vi "SnapToScore.vi"(7 "PigeonIMUDevRef":T1={"DeviceStatus"={"status"=FALSE, "code"=0, "source"=""}, "Device Number"=0, "Type"=352321536, "Device ID"=0, "Handle"=0, "UsageFrame"=0, "Library Path"=path ""} {"Type" items=["CAN"=352321536, "TalonSRX"=33554432]}, 11 "Robot Velocities In":cluster{"x":dbl, "y":dbl, "w":dbl}) -> (3 "Robot Velocities Out":cluster{"x":dbl, "y":dbl, "w":dbl})   [LabVIEW 2020]
uses:
  <vilib>/Rock Robotics/WPI/ThirdParty/Phoenix-LabVIEW/Pigeon IMU/CTRE_PigeonIMU_DeviceRef.ctl
  <vilib>/Rock Robotics/WPI/ThirdParty/Phoenix-LabVIEW/Pigeon IMU/CTRE_PigeonIMU_ConnectionType.ctl
  <vilib>/Analysis/coordinate.llb/Angle Range (Degree).ctl
  <vilib>/Analysis/coordinate.llb/Angle Units.ctl
  <vilib>/Analysis/_algsub.llb/Real Vector Norm.vi
  <vilib>/Analysis/coordinate.llb/Wrap Angle (scalar).vi
  <vilib>/Rock Robotics/WPI/ThirdParty/Phoenix-LabVIEW/Pigeon IMU/CTRE_PigeonIMU_GetYPR.vi
  <vilib>/Analysis/NI_AAL_Angle.lvlib
  <vilib>/Analysis/NI_AALPro.lvlib
panel:
  in  "Precision (deg)":dbl=0.25
  in  "static threshold":dbl=1.55
  in  "FEEEED":dbl=6.6
  out "Err/Out Chart":cluster{dbl, dbl}(graph)
  out "SP/PV Chart":cluster{"setpoint":dbl, "process variable":dbl}(graph)
  out "angle error":dbl
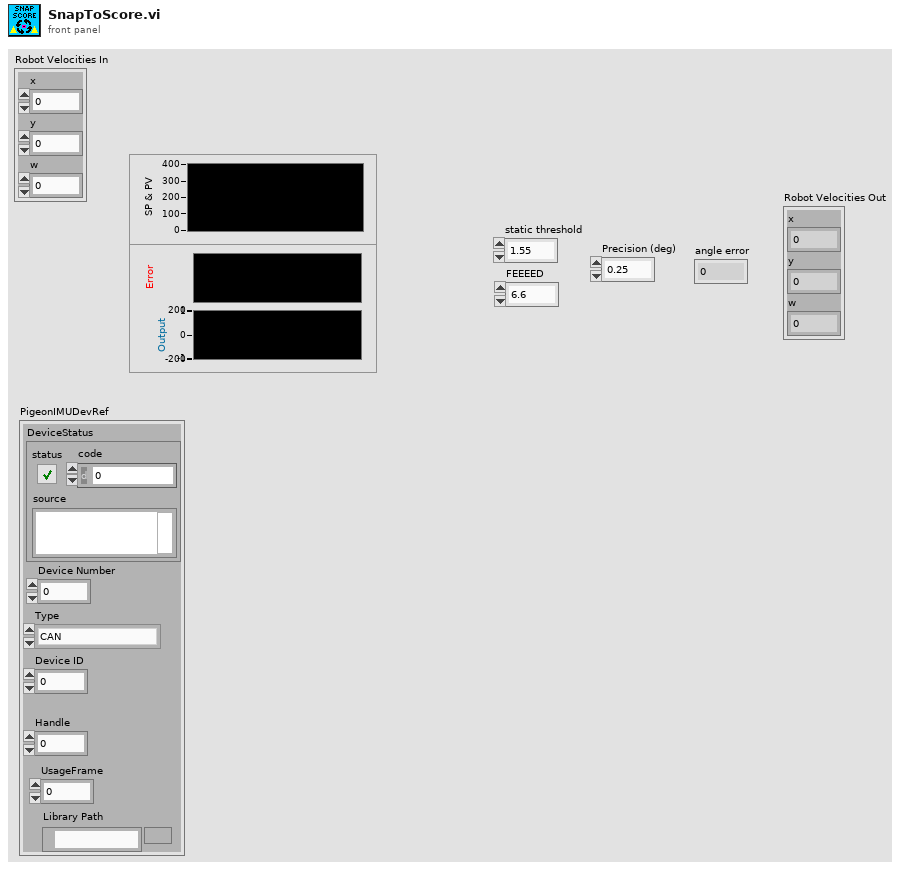
[diagram p1: front panel]
types:
  T1 = typedef "CTRE_PigeonIMU_DeviceRef.ctl" = cluster{"DeviceStatus":errorcluster, "Device Number":u8, "Type":T2, "Device ID":u32, "Handle":u64, "UsageFrame":u32, "Library Path":path}
  T2 = typedef "CTRE_PigeonIMU_ConnectionType.ctl" = u32
  T3 = cluster{"proportional gain (Kp)":dbl, "integral time (Ki)":dbl, "derivative time (Kd)":dbl}
  T4 = typedef "NI_AAL_Angle.lvlib/Angle Units.ctl" = i32
  T5 = typedef "NI_AAL_Angle.lvlib/Angle Range (Degree).ctl" = u16
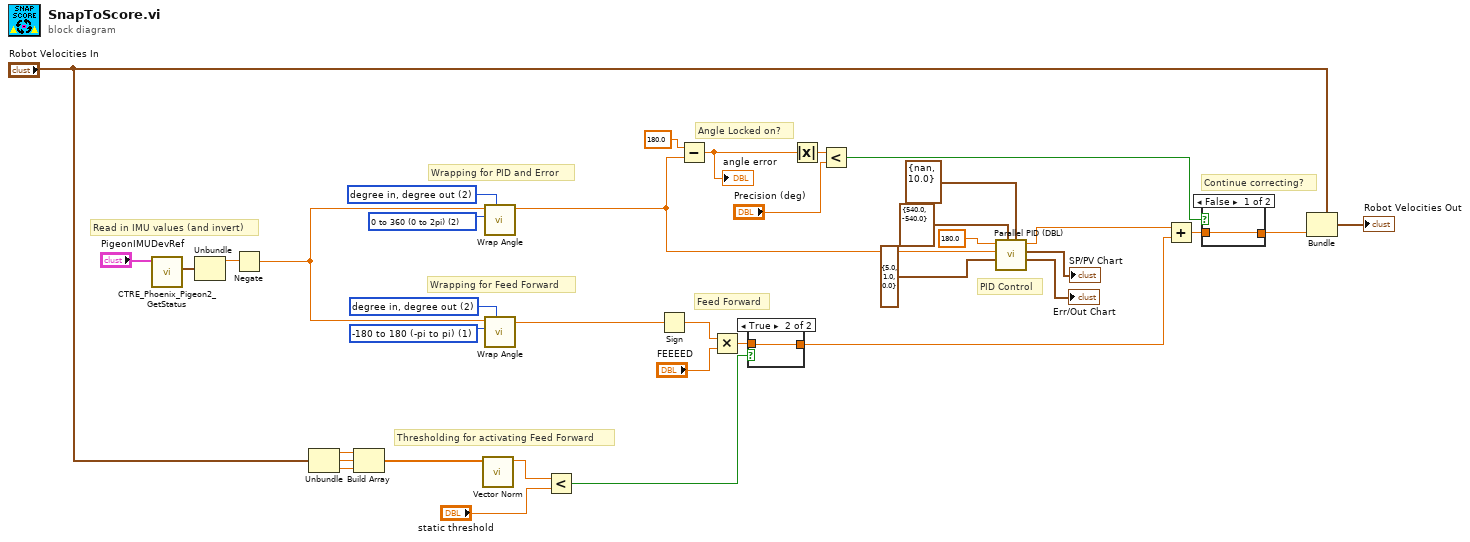
[diagram p0: block diagram]
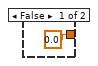
[diagram p2: hidden frame]
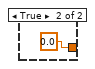
[diagram p3: hidden frame]
diagram:
  w21 = T4 2 items=["radian in, radian out", "radian in, degree out", "degree in, degree out", "degree in, radian out"] ("angle units")
  w24 = T5 1 items=["none", "-180 to 180 (-pi to pi)", "0 to 360 (0 to 2pi)"] ("angle range")
  w23 = T4 2 items=["radian in, radian out", "radian in, degree out", "degree in, degree out", "degree in, radian out"] ("angle units")
  w34 = T5 2 items=["none", "-180 to 180 (-pi to pi)", "0 to 360 (0 to 2pi)"] ("angle range")
  # "PID Control"
  # "Continue correcting?"
  # "Feed Forward"
  # "Angle Locked on?"
  # "Thresholding for activating Feed Forward"
  # "Read in IMU values (and invert)"
  # "Wrapping for Feed Forward"
  # "Wrapping for PID and Error"
  n1 = call-poly <vilib>:"CTRE_Phoenix_Pigeon2_GetStatus.vi"("PigeonIMUDevRef"="PigeonIMUDevRef") -> ("Yaw Pitch Roll"=w36:cluster{"Yaw":dbl, "Pitch":dbl, "Roll":dbl})  [unwired: 8 in, 2 out]
  n2 = Unbundle(w36) -> ("Yaw"=w26:dbl)  [unwired: 2 out]
  n3 = Negate(x=w26) -> (-x=w4:dbl)
  n4 = Unbundle("Robot Velocities In") -> ("x"=w19:dbl, "y"=w18:dbl, "w"=w16:dbl)
  n5 = Build Array(w19, w18, w16) -> (w17:dbl[])
  n6 = call-poly <vilib>:"Vector Norm.vi"("Input Vector"=w17) -> ("norm"=w15:dbl)  [unwired: 9 in, 1 out]
  n7 = call-poly <vilib>:"Wrap Angle.vi"("angle units"=w23, "angle range"=w34, "angle in"=w4) -> ("angle out"=w2:dbl)  [unwired: 7 in, 1 out]
  n8 = call-poly <vilib>:"Wrap Angle.vi"("angle units"=w21, "angle range"=w24, "angle in"=w4) -> ("angle out"=w22:dbl)  [unwired: 7 in, 1 out]
  n9 = Less?(x=w15, y="static threshold") -> (x < y?=w11:bool)
  n10 = Sign(1:w22) -> (0:w25:dbl)
  n11 = Subtract(x=180.0, y=w2) -> (x-y=w1:dbl)
  "angle error" <- w1
  n12 = Multiply(x=w25, y="FEEEED") -> (x*y=w13:dbl)
  n13 = case shown="True" w11 {
    tunnel: w13 -> [_ w39]
    tunnel: [0.0 w39] -> w12
    frame False {
    }
    frame True {
    }
  }
  n14 = Absolute Value(x=w1) -> (abs(x)=w9:dbl)
  n15 = Less?(x=w9, y="Precision (deg)") -> (x < y?=w7:bool)
  n16 = call <vilib>:"Parallel PID (DBL).vi"("advanced"=cluster{"alpha":dbl, "i-zone":dbl} {"alpha"=nan, "i-zone"=10.0}, "output range"=cluster{"high":dbl, "low":dbl} {"high"=540.0, "low"=-540.0}, "PID gains"=T3 {"proportional gain (Kp)"=5.0, "integral time (Ki)"=1.0, "derivative time (Kd)"=0.0}, "process variable"=w2, "setpoint"=180.0) -> ("Err/Out Chart"=→"Err/Out Chart":cluster{dbl, dbl}, "SP/PV Chart"=→"SP/PV Chart":cluster{"setpoint":dbl, "process variable":dbl}, "output"=w28:dbl)  [unwired: 3 in, 1 out]
  n17 = Add(x=w28, y=w12) -> (x+y=w6:dbl)
  n18 = case shown="False" w7 {
    tunnel: [w40 0.0] -> w5
    tunnel: w6 -> [w40 _]
    frame False {
    }
    frame True {
    }
  }
  n19 = Bundle(cluster="Robot Velocities In", "w"=w5) -> (→"Robot Velocities Out":cluster{"x":dbl, "y":dbl, "w":dbl})  [unwired: 2 in]
